vi "Interface_Asset_Map Control.vi"(8 "error in (no error)":errorcluster, 11 "EnergyStorage_Virtual in":refnum<class "EnergyStorage_Virtual.lvclass">) -> (0 "error out":errorcluster, 3 "EnergyStorage_Virtual out":refnum<class "EnergyStorage_Virtual.lvclass">)   [LabVIEW 2015, in "EnergyStorage_Virtual.lvclass"]
uses:
  EnergyStorage_Virtual.lvclass
panel:
  out "kW setpoint":dbl
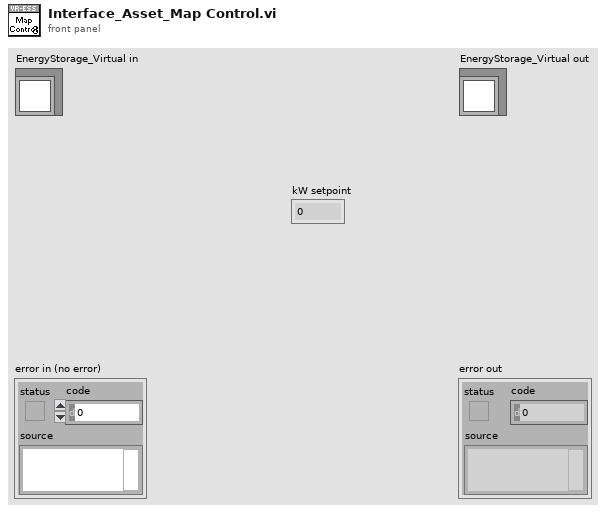
[diagram p1: front panel]
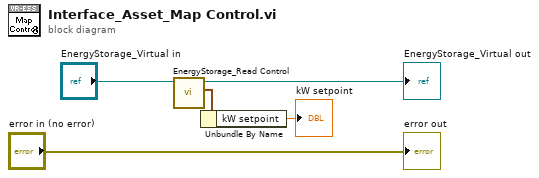
[diagram p0: block diagram]
diagram:
  n1 = call-dynamic "EnergyStorage_Read Control.vi"("EnergyStorage in"="EnergyStorage_Virtual in") -> ("EnergyStorage_Control"=w3:cluster{"kW setpoint":dbl}, "EnergyStorage out"=→"EnergyStorage_Virtual out":refnum<class "EnergyStorage_Virtual.lvclass">)  [unwired: 9 in]
  n2 = Unbundle By Name(w3) -> ("kW setpoint"=→"kW setpoint":dbl)
  "error out" <- "error in (no error)"
